vi "MathCad_String_Insert_to_Wrksht.vi"(3 "error out 2":errorcluster, 4 "New Variable Name":string, 5 "Mathcad.IStringValue":refnum<k7>, 6 "Worksheet Reference In":refnum<k7>) -> (0 "error out":errorcluster, 1 "Mathcad.IStringValue":refnum<k7>, 2 "Worksheet Reference Out":refnum<k7>)   [LabVIEW 2015]
doc: "Inserts value into the worksheet. This has to be done after the value has been set for the worksheet to recieve the new value."
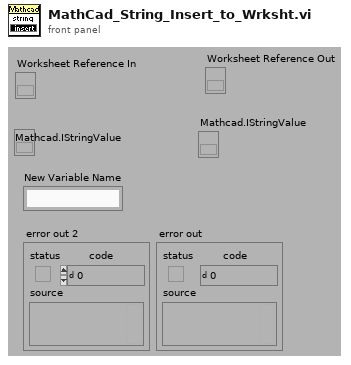
[diagram p1: front panel]
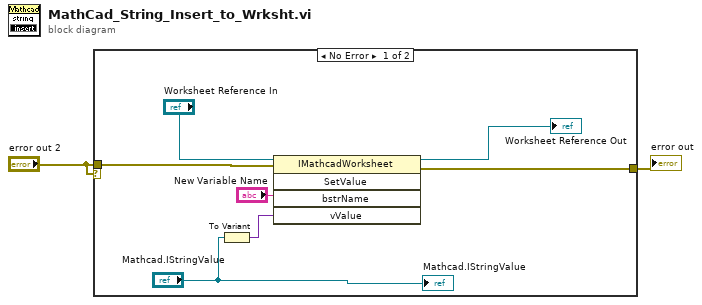
[diagram p0: block diagram]
diagram:
  n1 = case shown="No Error" "error out 2" {
    tunnel: [w9 w10] -> w2
    tunnel: "error out 2" -> [w6 w10]
    frame No Error {
      n2 = To Variant(anything="Mathcad.IStringValue") -> (Variant=w5:variant)
      n3 = invoke class="IMathcadWorksheet" method="SetValue"(reference="Worksheet Reference In", error in=w6, "bstrName"="New Variable Name", "vValue"=w5) -> (reference out=→"Worksheet Reference Out":refnum<k7>, error out=w9:errorcluster)  [unwired: 1 in, 3 out]
      "Mathcad.IStringValue" <- "Mathcad.IStringValue"
    }
    frame Error {
    }
  }
  "error out" <- w2
